vi "SynthHD_2_0a.vi"() -> ()   [LabVIEW 2012]
uses:
  Tab1.ctl
  <vilib>/Instr/_visa.llb/VISA Flush IO Buffer Mask.ctl
  <vilib>/Utility/file.llb/Read From Spreadsheet File (DBL).vi
  <vilib>/Utility/file.llb/Write To Spreadsheet File (DBL).vi
panel:
  out "RFOnB2":bool
  out "RFOnA2":bool
  out "Level B 2":bool
  out "Level A 2":bool
  in  "Modon":bool
  in  "Sync":bool
  out "POWER dBm B":dbl min=-100.0 max=24.0 step=1.0 format="%.2g"
  out "POWER dBm A":dbl min=-100.0 max=24.0 step=1.0 format="%.2g"
  out "RF  FREQUENCY MHz  B":dbl=1000.0 min=54.0 max=13900.0 step=1.0 format="%.7g"
  out "RF  FREQUENCY MHz A":dbl=1000.0 min=54.0 max=13900.0 step=1.0 format="%.7g"
  out "Amp Delta A -B":dbl format="%.2g"
  out "Freq Delta A-B":dbl format="%.7f"
  out "Device Under Control":string
  in  "AKNR":bool
  in  "PKNR":bool
  in  "FKNR":bool
  out "Channel":string="A"
  in  "ChSt":bool=TRUE
  out "COM Error":bool
  in  "Serial Port Select":refnum<visa-resource-name>="COM3"
  in  "stop":bool
  in  "Main Tab":T1
  in  "adn":bool
  in  "aup":bool
  in  "pdn":bool
  in  "pup":bool
  in  "fdn":bool
  in  "fup":bool
  out "Level":bool
  in  "Power Step Size":i32(ring)=3 items=["0.01dB", "0.05dB", "0.1 dB", "0.5 dB", "1.0 dB", "5.0 dB", "10.0 dB"]
  in  "RF  FREQUENCY MHz":dbl=1000.0 min=53.0 max=13999.999 step=1.0 format="%.7g"
  in  "Freqkn":i8(knob)=1 scale=1.0..20.0
  in  "Phasekn":i8(knob)=1 scale=1.0..20.0
  in  "PHASE Degrees":dbl min=0.0 max=360.0 step=1.0 format="%.2g"
  in  "POWER dBm":dbl min=-75.0 max=20.0 step=1.0 format="%.2g"
  in  "Powerkn":i8(knob)=1 scale=1.0..20.0
  in  "Frequency Step Size":i32(ring)=7 items=["0.1Hz", "1Hz", "10Hz", "100Hz", "1KHz", "10KHz", "100KHz", "1MHz", "10MHz", "100MHz", "1GHz"]
  in  "Phase Step Size":i32(ring)=6 items=["0.01 Degree", "0.05 Degree", "0.1 Degree", "0.5 Degree", "1 Degree", "5 Degree", "10 Degree", "90 Degree", "180 Degree"]
  in  "RF On":bool=TRUE
  in  "ChLock":bool
  in  "Sweep":enum32{"Linear", "List"}(tab)
  in  "Leveling":bool
  in  "Start Frequency":dbl=54.0 min=54.0 max=13900.0 step=0.001 format="%7.7f"
  in  "Step Size MHz":dbl=50.0 min=1e-07 max=13800.0 step=0.001 format="%.7f"
  in  "Stop Frequency":dbl=4000.0 min=54.0 max=13900.0 step=0.001 format="%7.7f"
  in  "Start Amplitude":dbl=22.0 min=-80.0 max=22.0 step=0.01 format="%7.2f"
  in  "Stop Amplitude":dbl=22.0 min=-80.0 max=22.0 step=0.01 format="%7.2f"
  out "Number\nof Points":u16
  out "Time per\nSweep (mS)":dbl format="%#.6g"
  in  "Read Table\nFrom File":bool
  in  "Save Table\nTo File":bool
  in  "Table RAM to\nTable NVROM":bool
  in  "Send Table\nTo RAM":bool
  in  "Sweep Table":dbl[][](array[numeric]) format="%#.6f"
  in  "Read Table\nFrom Device":bool
  in  "sweepdiff":bool
  in  "Sweep\nOnce":bool
  in  "Sweep\nContinuously":bool
  in  "sweepdir":bool
  in  "Differential Freq":dbl=54.0 min=-13800.0 max=13800.0 step=0.001 format="%7.7f"
  in  "Step Time (mS)":dbl=4.0 min=4.0 max=10000.0 step=0.001 format="%.3f"
  out "Swpc":string
  in  "Mod Tab":enum32{"PULSE Amplitude", "AM", "FM"}(tab)
  in  "Dual Channel Mode":bool
  in  "Send Pulse\nBurst":bool
  out "Duration (uS)":dbl
  in  "Continuous\nPM":bool
  in  "# of Pulses in Burst":u16=100 min=1 max=65500 step=1 format="%#.5f"
  in  "Off Time (uS)":u32=10 min=2 max=10000000 step=1
  in  "On Time (uS)":u32=1 max=10000000 step=1
  out "Pulsech":string
  in  "Invert\nPulse":bool
  in  "Read AM":bool
  out "Samples/Cycle":u8
  in  "Save AM to ROM":bool
  out "AMch":string
  in  "AM Freq (Hz)":dbl=500.0 min=1.0 max=5000.0 step=1.0 format="%.2f"
  out "Actual Freq (Hz)":dbl
  in  "Peak Power(dBm)":dbl=15.0 min=-74.9 max=20.0 step=0.01 format="%.2f"
  in  "Minimum Power (dBm)":dbl=15.0 min=-74.9 max=20.0 step=0.01 format="%.2f"
  in  "Continuous AM":bool
  in  "Wave Shape":u8(ring) items=["Sine", "Ramp", "Triangle"]
  out "Waveform":dbl[](graph)
  in  "Linear in?":u8(ring) items=["Linear in dB", "Linear in Volts"]
  in  "AM Samples in Burst":u16=100 min=1 max=5000 step=1 format="%#.5f"
  in  "FM Rate (Hz)":u16=500 min=1 max=5000 step=1
  in  "FM Deviation (+/- Hz)":u32=500 min=10 step=1
  in  "Continuous FM":bool
  in  "FM Samples in Burst":u16=100 min=1 max=65500 step=1 format="%#.5f"
  out "FMch":string
  in  "FM Function":u8(ring) items=["Sine", "Chirp"]
  out "FM Samples / Cycle":u16
  out "Specific Instructions":string
  in  "Trigger":i32(ring) items=["No Triggers", "Full Frequency Sweep", "Single Sweep Step", "Stop All", "Digital RF On/Off", "Remove Interrupts", "Reserved 1", "Reserved 2", "Ext AM Modulation", "Ext FM Modulation"]
  in  "Read Registers":bool
  in  "Read Settings\nFrom SynthHD":bool
  out "read buffer":string
  out "Hex buf":string
  in  "MUX Out Select":u8(ring)=6 items=["HiZ", "Vdd", "GND", "R Divider", "N Divider", "An Lock Det", "Dig Lock Det"]
  in  "PLL ICP":u8=4 max=15 step=1 format="%02d"
  out "HW Version":string
  in  "Get Phase\nLock Status":bool
  out "FW Version":string
  in  "Read\nVersion":bool
  in  "Save Settings\nto ROM":bool
  in  "Get\nTemperature":bool
  out "Temperature":string
  in  "Fundamental\nFeedback Mode":bool
  out "Lock":bool
  in  "MTLD":bool
  in  "Re-Init Settings\nto Default":bool
  in  "Reference Select":u8(ring)=1 items=["External", "Internal 27MHz", "Internal 10MHz"]
  in  "Reference (MHz)":dbl=27.0 min=5.0 max=111.0 step=0.001 format="%7.6g"
  # "A"
  # "B"
  # "v2.0a"
  # "Windfreak Technologies"
  # "A"
  # "B"
  # "Tab selection dictates sweep mode"
  # "Step"
  # "Freq(MHz)"
  # "Level(dBm)"
  # "Burst"
  # "Widest FM Deviation+/- \n54-106.25MHz = 160KHz\n-212.5MHz        = 312KHz\n-425.0MHz        = 625KHz\n-850.0MHz      = 1.25MHz\n-1700MHz         = 2.5MHz\n-3400MHz            = 5MHz\n-6800MHz          = 10MHz\n-13600MHz        = 20MHz"
  # "Digital Trigger 0V to +3.3V only.\nAnalog Input 0V to 1.2V only.\nTrigger has ~35K ohm pullup\nfor both modes."
  # "C"
  # "Windfreak Technologies, LLC 2015"
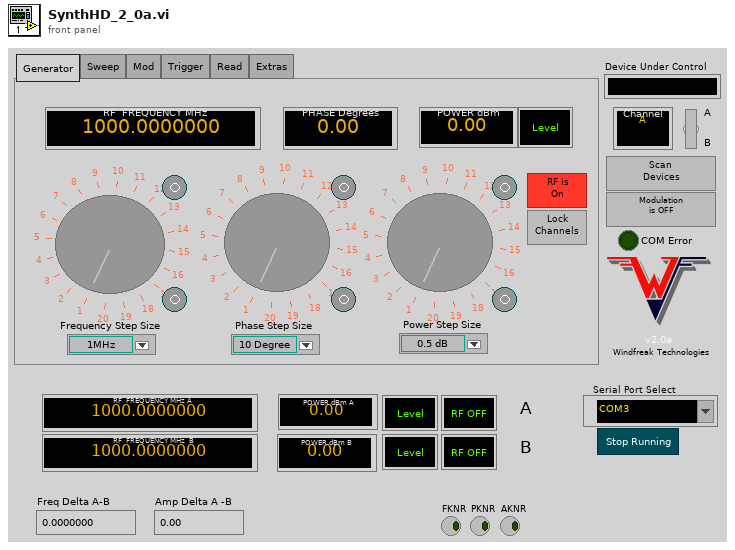
[diagram p1: front panel]
types:
  T1 = typedef "Tab1.ctl" = enum32{"Generator", "Sweep", "Mod", "Trigger", "Read", "Extras"}
  T2 = enum8{"Enabled", "Disabled", "Disabled and Grayed Out"}
  T3 = cluster{"[0]":dbl, "[1]":dbl, "[2]":dbl, "[3]":dbl, "[4]":dbl, "[5]":dbl, "[6]":dbl, "[7]":dbl, "[8]":dbl, "[9]":dbl, "[10]":dbl, "[11]":dbl, "[12]":dbl, "[13]":dbl, "[14]":dbl, "[15]":dbl, "[16]":dbl, "[17]":dbl, "[18]":dbl, "[19]":dbl, "[20]":dbl, "[21]":dbl, "[22]":dbl, "[23]":dbl, "[24]":dbl, "[25]":dbl, "[26]":dbl, "[27]":dbl, "[28]":dbl, "[29]":dbl, "[30]":dbl, "[31]":dbl, "[32]":dbl, "[33]":dbl, "[34]":dbl, "[35]":dbl, "[36]":dbl, "[37]":dbl, "[38]":dbl, "[39]":dbl, "[40]":dbl, "[41]":dbl}
  T4 = typedef "VISA Flush IO Buffer Mask.ctl" = u16
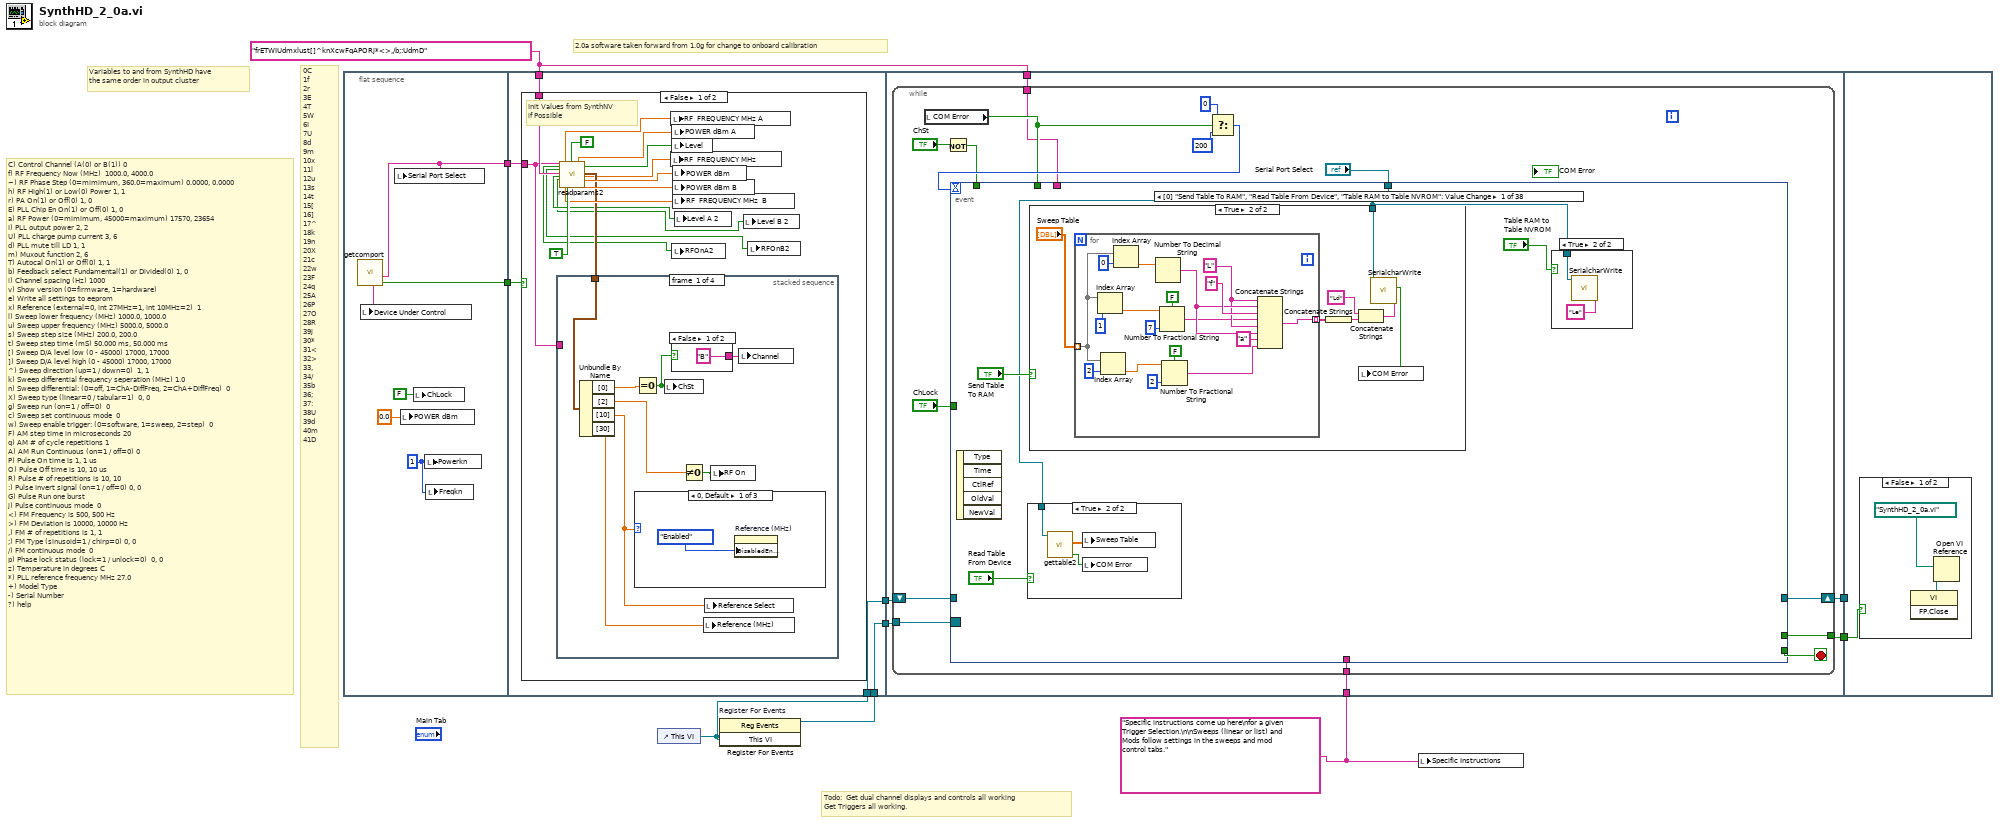
[diagram p0: block diagram]
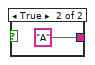
[diagram p2: hidden frame]
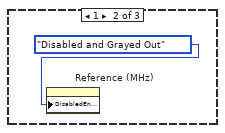
[diagram p3: hidden frame]
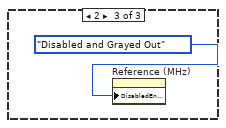
[diagram p4: hidden frame]
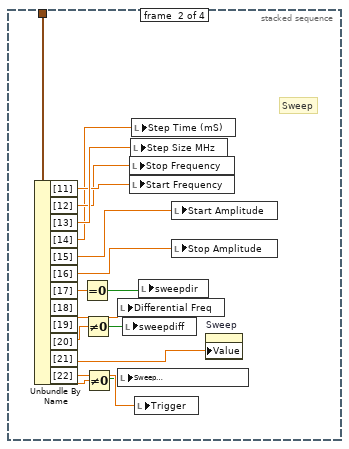
[diagram p5: hidden frame]
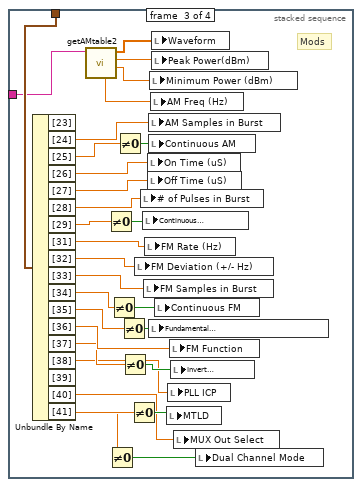
[diagram p6: hidden frame]
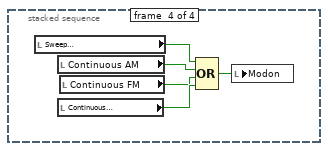
[diagram p7: hidden frame]
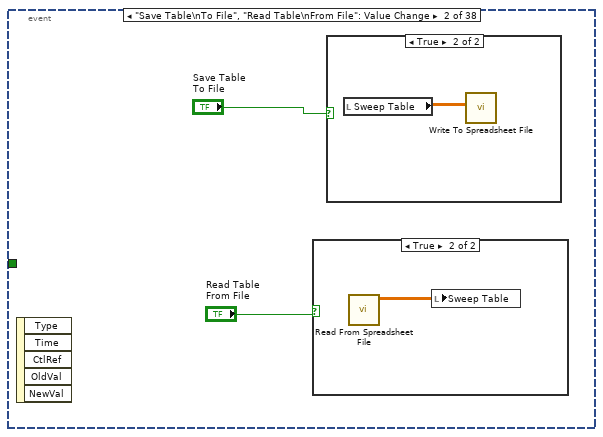
[diagram p12: hidden frame]
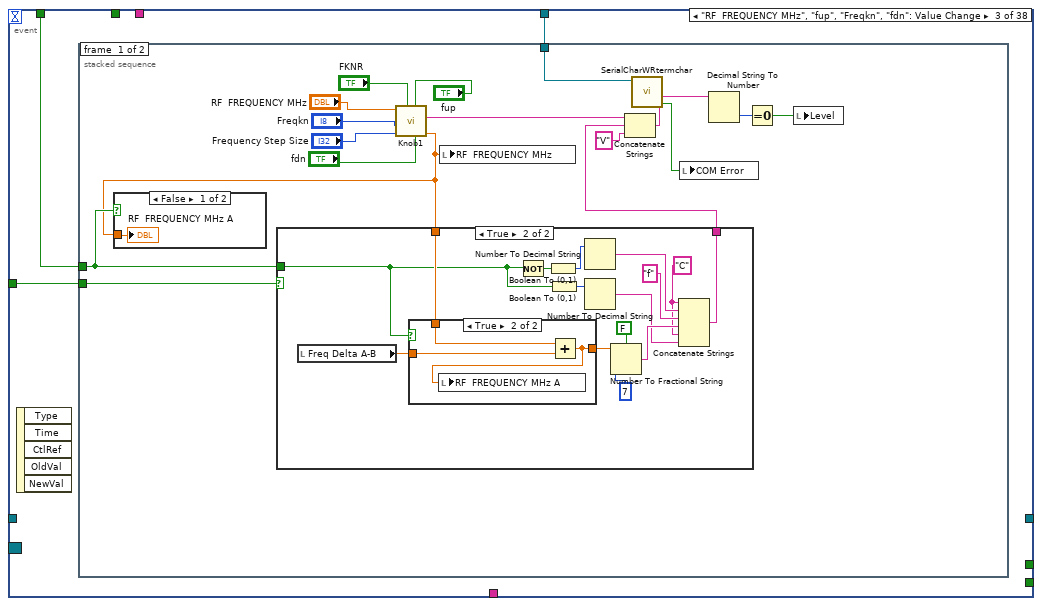
[diagram p15: hidden frame]
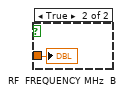
[diagram p16: hidden frame]
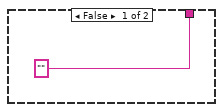
[diagram p17: hidden frame]
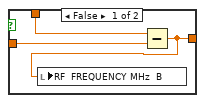
[diagram p18: hidden frame]
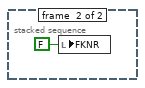
[diagram p19: hidden frame]
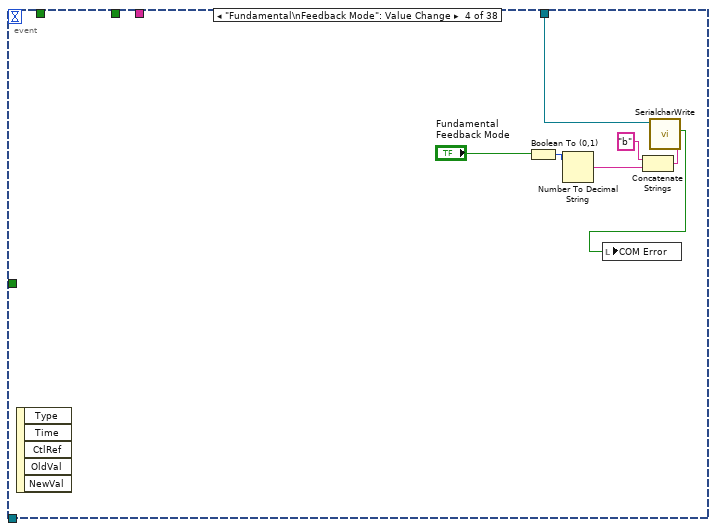
[diagram p20: hidden frame]
diagram:
  w1 = "Specific instructions come up here\nfor a given Trigger Selection.\n\nSweeps (linear or list) and Mods follow settings in the sweeps and mod control tabs." ("message")
  w4 = "frETWIUdmxlust[]^knXcwFqAPORj*<>,/b;:UdmD" ("var query")
  # "Todo:  Get dual channel displays and controls all working\nGet Triggers all working."
  # "2.0a software taken forward from 1.0g for change to onboard calibration"
  # "C) Control Channel (A(0) or B(1)) 0\nf) RF Frequency Now (MHz)  1000.0, 4000.0\n~) RF Phase Step (0=mimimum, 360.0=maximum) 0.0000, 0.0000\nh) RF High(1) or Low(0) Power 1, 1\nr) PA On(1) or Off(0) 1, 0\nE) PLL Chip En On(1) or Off(0) 1, 0\na) RF Power (0=mimimum, 45000=maximum) 17570, 23654\nI) PLL output power 2, 2\nU) PLL charge pump current 3, 6\nd) PLL mute till LD 1, 1\nm) Muxout function 2, 6\nT) Autocal On(1) or Off(0) 1, 1\nb) Feedback select Fundamental(1) or Divided(0) 1, 0\ni) Channel spacing (Hz) 1000\nv) Show version (0=firmware, 1=hardware)\ne) Write all settings to eeprom\nx) Reference (external=0, int 27MHz=1, int 10MHz=2)  1\nl) Sweep lower frequency (MHz) 1000.0, 1000.0\nu) Sweep upper frequency (MHz) 5000.0, 5000.0\ns) Sweep step size (MHz) 200.0, 200.0\nt) Sweep step time (mS) 50.000 ms, 50.000 ms\n[) Sweep D/A level low (0 - 45000) 17000, 17000\n]) Sweep D/A level high (0 - 45000) 17000, 17000\n^) Sweep direction (up=1 / down=0)  1, 1\nk) Sweep differential frequency seperation (MHz) 1.0\nn) Sweep differential: (0=off, 1=ChA-DiffFreq, 2=ChA+DiffFreq)  0\nX) Sweep type (linear=0 / tabular=1)  0, 0\ng) Sweep run (on=1 / off=0)  0\nc) Sweep set continuous mode  0\nw) Sweep enable trigger: (0=software, 1=sweep, 2=step)  0\nF) AM step time in microseconds 20\nq) AM # of cycle repetitions 1\nA) AM Run Continuous (on=1 / off=0) 0\nP) Pulse On time is 1, 1 us\nO) Pulse Off time is 10, 10 us\nR) Pulse # of repetitions is 10, 10\n:) Pulse Invert signal (on=1 / off=0) 0, 0\nG) Pulse Run one burst\nj) Pulse continuous mode  0\n<) FM Frequency is 500, 500 Hz\n>) FM Deviation is 10000, 10000 Hz\n,) FM # of repetitions is 1, 1\n;) FM Type (sinusoid=1 / chirp=0) 0, 0\n/) FM continuous mode  0\np) Phase lock status (lock=1 / unlock=0)  0, 0\nz) Temperature in degrees C\n*) PLL reference frequency MHz 27.0\n+) Model Type\n-) Serial Number  \n?) help"
  # "0C\n1f\n2r\n3E\n4T\n5W\n6I\n7U\n8d\n9m\n10x\n11l\n12u\n13s\n14t\n15[\n16]\n17^\n18k\n19n\n20X\n21c\n22w\n23F\n24q\n25A\n26P\n27O\n28R\n39j\n30*\n31<\n32>\n33,\n34/\n35b\n36;\n37:\n38U\n39d\n40m\n41D"
  # "Variables to and from SynthHD have \nthe same order in output cluster"
  n1 = flat-sequence {
    tunnel: [w16] -> w10
    tunnel: [w15] -> w9
    tunnel: w10 -> [w21]
    tunnel: w9 -> [w20]
    tunnel: [w18] -> w8
    tunnel: [w17] -> w7
    tunnel: w4 -> [w19]
    tunnel: w3 -> [w18]
    tunnel: w2 -> [w17]
    tunnel: w8 -> [w106]
    tunnel: w7 -> [w107]
    tunnel: [w105] -> w6
    tunnel: [w104] -> w5
    tunnel: w4 -> [w103]
    tunnel: w1 -> [w102]
    tunnel: w6 -> [_]
    tunnel: w5 -> [w811]
    frame #0 {
      w13 = i8 1 ("Powerkn")
      n2 = call "getcomport.vi"() -> ("No Devices"=w16:bool, "Port"=w15:string, "Device"=w14:string)  [unwired: 9 in]
      n3 = local write "Device Under Control"(w14) -> ()
      n4 = local write "Serial Port Select"(w15) -> ()
      n5 = local write "POWER dBm"(0.0 ("Power")) -> ()
      n6 = local write "ChLock"(FALSE ("ChLock")) -> ()
      n7 = local write "Powerkn"(w13) -> ()
      n8 = local write "Freqkn"(w13) -> ()
    }
    frame #1 {
      n9 = case shown="False" w21 {
        tunnel: w20 -> [w27 _]
        tunnel: w19 -> [w37 _]
        frame False {
          # "Init Values from SynthNV\nif Possible"
          n10 = call "readparams2.vi"("Port In"=w27, "var query"=w37, "Get F&A"=TRUE, "Prog Chan?"=FALSE) -> ("RFonA"=w23:bool, "RFonB"=w22:bool, "LevA"=w25:bool, "LevB"=w24:bool, "FchA"=w35:dbl, "FchB"=w32:dbl, "AdBm"=w34:dbl, "BdBm"=w33:dbl, "NowLevel"=w31:bool, "cluster"=w28:T3, "NowFreq"=w26:dbl, "NowdBm"=w30:dbl)  [unwired: 9 in, 3 out]
          n11 = stacked-sequence {
            tunnel: w28 -> [w42 w66 w96 _]
            tunnel: w27 -> [_ _ w84 _]
            frame #0 {
              n12 = Unbundle By Name(w42) -> ("[0]"=w45:dbl, "[2]"=w44:dbl, "[10]"=w41:dbl, "[30]"=w40:dbl)
              n13 = Equal To 0?(x=w45) -> (x = 0?=w38:bool)
              n14 = case shown="0, Default" w41 {
                frame 0, Default {
                  n15 = property on="Reference (MHz)" class="DigNum (strict)"("DisabledEnum"=T2."Enabled" ("Disabled")) -> ()  [unwired: 2 in, 2 out]
                }
                frame 1 {
                  n16 = property on="Reference (MHz)" class="DigNum (strict)"("DisabledEnum"=T2."Disabled and Grayed Out" ("Disabled")) -> ()  [unwired: 2 in, 2 out]
                }
                frame 2 {
                  n17 = property on="Reference (MHz)" class="DigNum (strict)"("DisabledEnum"=T2."Disabled and Grayed Out" ("Disabled")) -> ()  [unwired: 2 in, 2 out]
                }
              }
              n18 = local write "ChSt"(w38) -> ()
              n19 = case shown="False" w38 {
                tunnel: ["B" ("Channel") "A" ("Channel")] -> w43
                frame False {
                }
                frame True {
                }
              }
              n20 = Not Equal To 0?(x=w44) -> (x != 0?=w39:bool)
              n21 = local write "Reference (MHz)"(w40) -> ()
              n22 = local write "Reference Select"(w41) -> ()
              n23 = local write "RF On"(w39) -> ()
              n24 = local write "Channel"(w43) -> ()
            }
            frame #1 {
              # "Sweep"
              n25 = Unbundle By Name(w66) -> ("[11]"=w56:dbl, "[12]"=w55:dbl, "[13]"=w65:dbl, "[14]"=w54:dbl, "[15]"=w52:dbl, "[16]"=w51:dbl, "[17]"=w64:dbl, "[18]"=w62:dbl, "[19]"=w61:dbl, "[20]"=w57:dbl, "[21]"=w53:dbl, "[22]"=w59:dbl)
              n26 = Equal To 0?(x=w64) -> (x = 0?=w63:bool)
              n27 = Not Equal To 0?(x=w61) -> (x != 0?=w60:bool)
              n28 = Not Equal To 0?(x=w53) -> (x != 0?=w58:bool)
              n29 = local write "Differential Freq"(w62) -> ()
              n30 = local write "Sweep\nContinuously"(w58) -> ()
              n31 = local write "sweepdiff"(w60) -> ()
              n32 = local write "Stop Frequency"(w55) -> ()
              n33 = local write "Start Frequency"(w56) -> ()
              n34 = local write "Step Size MHz"(w65) -> ()
              n35 = local write "Step Time (mS)"(w54) -> ()
              n36 = local write "Trigger"(w59) -> ()
              n37 = local write "sweepdir"(w63) -> ()
              n38 = local write "Start Amplitude"(w52) -> ()
              n39 = local write "Stop Amplitude"(w51) -> ()
              n40 = property on="Sweep" class="TabCtl (strict)"("Value"=w57) -> ()  [unwired: 2 in, 2 out]
            }
            frame #2 {
              # "Mods"
              n41 = Unbundle By Name(w96) -> ("[24]"=w81:dbl, "[25]"=w93:dbl, "[26]"=w92:dbl, "[27]"=w91:dbl, "[28]"=w90:dbl, "[29]"=w89:dbl, "[31]"=w83:dbl, "[32]"=w82:dbl, "[33]"=w79:dbl, "[34]"=w80:dbl, "[35]"=w76:dbl, "[36]"=w75:dbl, "[37]"=w73:dbl, "[38]"=w72:dbl, "[39]"=w70:dbl, "[40]"=w69:dbl, "[41]"=w68:dbl)  [unwired: 1 out]
              n42 = call "getAMtable2.vi"("Serial Port Select"=w84) -> ("Min dB"=w85:dbl, "Max dB"=w86:dbl, "Waveform Graph"=w87:dbl[], "AM Freq Hz"=w88:dbl)  [unwired: 5 in, 2 out]
              n43 = Not Equal To 0?(x=w89) -> (x != 0?=w94:bool)
              n44 = Not Equal To 0?(x=w68) -> (x != 0?=w67:bool)
              n45 = Not Equal To 0?(x=w80) -> (x != 0?=w78:bool)
              n46 = Not Equal To 0?(x=w93) -> (x != 0?=w95:bool)
              n47 = Not Equal To 0?(x=w76) -> (x != 0?=w77:bool)
              n48 = Not Equal To 0?(x=w73) -> (x != 0?=w74:bool)
              n49 = Not Equal To 0?(x=w70) -> (x != 0?=w71:bool)
              n50 = local write "FM Deviation (+/- Hz)"(w82) -> ()
              n51 = local write "# of Pulses in Burst"(w90) -> ()
              n52 = local write "Continuous\nPM"(w94) -> ()
              n53 = local write "FM Samples in Burst"(w79) -> ()
              n54 = local write "FM Rate (Hz)"(w83) -> ()
              n55 = local write "On Time (uS)"(w92) -> ()
              n56 = local write "Off Time (uS)"(w91) -> ()
              n57 = local write "AM Samples in Burst"(w81) -> ()
              n58 = local write "Continuous AM"(w95) -> ()
              n59 = local write "Fundamental\nFeedback Mode"(w77) -> ()
              n60 = local write "Minimum Power (dBm)"(w85) -> ()
              n61 = local write "AM Freq (Hz)"(w88) -> ()
              n62 = local write "Waveform"(w87) -> ()
              n63 = local write "Peak Power(dBm)"(w86) -> ()
              n64 = local write "Continuous FM"(w78) -> ()
              n65 = local write "MTLD"(w71) -> ()
              n66 = local write "PLL ICP"(w72) -> ()
              n67 = local write "FM Function"(w75) -> ()
              n68 = local write "Invert\nPulse"(w74) -> ()
              n69 = local write "MUX Out Select"(w69) -> ()
              n70 = local write "Dual Channel Mode"(w67) -> ()
            }
            frame #3 {
              n71 = local read "Sweep\nContinuously"() -> (w98:bool)
              n72 = local read "Continuous AM"() -> (w99:bool)
              n73 = local read "Continuous\nPM"() -> (w101:bool)
              n74 = local read "Continuous FM"() -> (w100:bool)
              n75 = Compound Arithmetic op=OR(w98, w99, w100, w101) -> (w97:bool)
              n76 = local write "Modon"(w97) -> ()
            }
          }
          n77 = local write "RF  FREQUENCY MHz A"(w35) -> ()
          n78 = local write "RF  FREQUENCY MHz"(w26) -> ()
          n79 = local write "POWER dBm A"(w34) -> ()
          n80 = local write "Level"(w31) -> ()
          n81 = local write "RFOnA2"(w23) -> ()
          n82 = local write "POWER dBm"(w30) -> ()
          n83 = local write "POWER dBm B"(w33) -> ()
          n84 = local write "RF  FREQUENCY MHz  B"(w32) -> ()
          n85 = local write "Level A 2"(w25) -> ()
          n86 = local write "Level B 2"(w24) -> ()
          n87 = local write "RFOnB2"(w22) -> ()
        }
        frame True {
        }
      }
    }
    frame #2 {
      n88 = while {
        shift-right: [w118] -> w105
        shift-left: w107 -> [w120]
        tunnel: w106 -> [w119]
        tunnel: [w117] -> w104
        tunnel: w103 -> [w112]
        tunnel: w102 -> [w108]
        stop <- w121 stop-if-true
        n89 = local read "COM Error"() -> (w113:bool)
        n90 = Not(x="ChSt") -> (.not. x?=w110:bool)
        n91 = Select(t=0, s=w113, f=200) -> (s? t:f=w114:i32)
        n92 = event shown="[0] \"Send Table To RAM\", \"Read Table From Device\", \"Table RAM to Table NVROM\": Value Change" {
          selector: w119 -> [_ _ _ _ _ _ _ _ _ _ _ _ _ _ _ _ _ _ _ _ _ _ _ _ _ _ _ _ _ _ _ _ _ _ _ _ _ _]
          dyn-events: _ -> [_ _ _ _ _ _ _ _ _ _ _ _ _ _ _ _ _ _ _ _ _ _ _ _ _ _ _ _ _ _ _ _ _ _ _ _ _ _]
          timeout: w114 -> [_ _ _ _ _ _ _ _ _ _ _ _ _ _ _ _ _ _ _ _ _ _ _ _ _ _ _ _ _ _ _ _ _ _ _ _ _ _]
          tunnel: "Serial Port Select" -> [w123 _ w163 w207 w214 w254 w326 _ w374 w403 w425 w437 w471 w479 w496 w509 w524 w539 w542 w544 w549 w552 w560 w564 w585 w589 w594 w601 w718 w751 w764 w771 w775 _ _ w784 w790 w800]
          tunnel: [_ _ _ _ _ _ _ _ _ _ _ _ _ _ _ _ _ _ _ _ _ _ _ _ _ _ _ _ _ _ _ _ _ "stop" w781 _ _ _] -> w121
          tunnel: w120 -> [_ _ _ _ _ _ _ _ _ _ _ _ _ _ _ _ _ _ _ _ _ _ _ _ _ _ _ _ _ _ _ _ _ _ w780 _ _ _]
          tunnel: [_ _ _ _ _ _ _ _ _ _ _ _ _ _ _ _ _ _ _ _ _ _ _ _ _ _ _ _ _ _ _ _ _ _ w780 _ _ _] -> w118
          tunnel: [_ _ _ _ _ _ _ _ _ _ _ _ _ _ _ _ _ _ _ _ _ _ _ _ _ _ _ _ _ _ _ _ _ "stop" _ _ _ _] -> w117
          tunnel: w113 -> [_ _ _ _ _ _ _ _ _ _ _ _ _ _ _ _ _ _ _ _ _ _ _ _ _ _ _ _ _ _ _ _ _ _ _ w783 _ _]
          tunnel: w112 -> [_ _ _ _ _ _ _ _ _ _ _ _ _ _ _ _ _ _ _ _ _ _ _ _ _ _ _ w602 _ _ _ _ _ _ _ _ _ _]
          tunnel: w110 -> [_ _ w162 _ _ w253 w319 _ _ _ _ w435 w463 _ w489 _ w518 _ _ _ _ _ _ _ _ _ _ w600 _ _ w755 _ _ _ _ _ _ _]
          tunnel: "ChLock" -> [_ _ w161 _ _ w252 _ _ _ _ _ _ _ _ _ _ _ _ _ _ _ _ _ _ _ _ _ _ _ _ _ _ _ _ _ _ _ _]
          tunnel: w108 -> [_ _ _ _ _ _ _ _ _ w400 _ _ _ _ _ _ _ _ _ _ _ _ _ _ _ _ _ _ _ _ _ _ _ _ _ _ _ _]
          event "Send Table\nTo RAM", "Read Table\nFrom Device", "Table RAM to\nTable NVROM": Value Change {
            n93 = event-data() -> ()  [unwired: 1 in, 5 out]
            n94 = case shown="True" "Read Table\nFrom Device" {
              tunnel: w123 -> [_ w131]
              frame False {
              }
              frame True {
                n95 = call "gettable2.vi"("Serial Port Select"=w131) -> ("COM Error"=w130:bool, "Sweep Table"=w129:dbl[][])  [unwired: 9 in]
                n96 = local write "Sweep Table"(w129) -> ()
                n97 = local write "COM Error"(w130) -> ()
              }
            }
            n98 = case shown="True" "Send Table\nTo RAM" {
              tunnel: w123 -> [_ w137]
              frame False {
              }
              frame True {
                n99 = for {
                  tunnel: "Sweep Table" -> [w145] mode=indexing
                  tunnel: [w151] -> w132 mode=indexing
                  w148 = "L" ("string")
                  n100 = Index Array(array=w145, index=1) -> (element=w144:dbl)
                  n101 = Index Array(array=w145, index=2) -> (element=w140:dbl)
                  n102 = Index Array(array=w145, index=0) -> (element=w149:dbl)
                  n103 = Number To Decimal String(number=w149) -> (decimal integer string=w152:string)  [unwired: 1 in]
                  n104 = Number To Fractional String(use system decimal point (T)=FALSE, number=w144, precision (6)=i16 7) -> (F-format string=w147:string)  [unwired: 1 in]
                  n105 = Number To Fractional String(use system decimal point (T)=FALSE, number=w140, precision (6)=i16 2) -> (F-format string=w139:string)  [unwired: 1 in]
                  n106 = Concatenate Strings(w148, w152, "f" ("string"), w147, w148, w152, "a" ("string"), w139) -> (w151:string)
                }
                n107 = Concatenate Strings(w132) -> (w135:string)
                n108 = Concatenate Strings("Ld" ("string"), w135) -> (w133:string)
                n109 = call "SerialcharWrite.vi"("VISA resource name"=w137, "write buffer"=w133) -> ("ComError"=w136:bool)  [unwired: 8 in]
                n110 = local write "COM Error"(w136) -> ()
              }
            }
            n111 = case shown="True" "Table RAM to\nTable NVROM" {
              tunnel: w123 -> [_ w128]
              frame False {
              }
              frame True {
                n112 = call "SerialcharWrite.vi"("VISA resource name"=w128, "write buffer"="Le") -> ()  [unwired: 8 in, 1 out]
              }
            }
          }
          event "Save Table\nTo File", "Read Table\nFrom File": Value Change {
            n113 = event-data() -> ()  [unwired: 1 in, 5 out]
            n114 = case shown="True" "Read Table\nFrom File" {
              frame False {
              }
              frame True {
                n115 = call-poly <vilib>:"Read From Spreadsheet File.vi"() -> ("all rows"=w159:dbl[][])  [unwired: 7 in, 4 out]
                n116 = local write "Sweep Table"(w159) -> ()
              }
            }
            n117 = case shown="True" "Save Table\nTo File" {
              frame False {
              }
              frame True {
                n118 = local read "Sweep Table"() -> (w160:dbl[][])
                n119 = call-poly <vilib>:"Write To Spreadsheet File.vi"("2D data"=w160) -> ()  [unwired: 7 in, 1 out]
              }
            }
          }
          event "RF  FREQUENCY MHz", "fup", "Freqkn", "fdn": Value Change {
            n120 = event-data() -> ()  [unwired: 1 in, 5 out]
            n121 = stacked-sequence {
              tunnel: w163 -> [w181 _]
              tunnel: w162 -> [w169 _]
              tunnel: w161 -> [w171 _]
              frame #0 {
                n122 = call "Knob1.vi"("Freqin"="RF  FREQUENCY MHz", "Knob"="Freqkn", "Frequency Step Size"="Frequency Step Size", "Reset"="FKNR", "fup"="fup", "fdn"="fdn") -> ("freqcommand"=w176:string, "freqout"=w168:dbl)  [unwired: 3 in]
                n123 = case shown="False" w169 {
                  tunnel: w168 -> [w182 w183]
                  frame False {
                    "RF  FREQUENCY MHz A" <- w182
                  }
                  frame True {
                    "RF  FREQUENCY MHz  B" <- w183
                  }
                }
                n124 = case shown="True" w171 {
                  tunnel: ["" ("string") w199] -> w170
                  tunnel: w168 -> [_ w190]
                  tunnel: w169 -> [_ w187]
                  frame False {
                  }
                  frame True {
                    w186 = "C" ("string")
                    n125 = local read "Freq Delta A-B"() -> (w192:dbl)
                    n126 = case shown="True" w187 {
                      tunnel: w190 -> [w201 w205]
                      tunnel: [w200 w203] -> w189
                      tunnel: w192 -> [w202 w204]
                      frame False {
                        n127 = Subtract(x=w201, y=w202) -> (x-y=w200:dbl)
                        n128 = local write "RF  FREQUENCY MHz  B"(w200) -> ()
                      }
                      frame True {
                        n129 = Add(x=w205, y=w204) -> (x+y=w203:dbl)
                        n130 = local write "RF  FREQUENCY MHz A"(w203) -> ()
                      }
                    }
                    n131 = Not(x=w187) -> (.not. x?=w188:bool)
                    n132 = Boolean To (0,1)(Boolean=w188) -> (0, 1=w194:i16)
                    n133 = Boolean To (0,1)(Boolean=w187) -> (0, 1=w193:i16)
                    n134 = Number To Decimal String(number=w194) -> (decimal integer string=w198:string)  [unwired: 1 in]
                    n135 = Number To Decimal String(number=w193) -> (decimal integer string=w185:string)  [unwired: 1 in]
                    n136 = Number To Fractional String(use system decimal point (T)=FALSE, number=w189, precision (6)=i16 7) -> (F-format string=w195:string)  [unwired: 1 in]
                    n137 = Concatenate Strings(w186, w198, "f" ("string"), w195, w186, w185) -> (w199:string)
                  }
                }
                n138 = local write "RF  FREQUENCY MHz"(w168) -> ()
                n139 = Concatenate Strings(w176, w170, "V" ("string")) -> (w179:string)
                n140 = call "SerialCharWRtermchar.vi"("VISA resource name"=w181, "write buffer"=w179) -> ("error?"=w180:bool, "read buffer"=w164:string)  [unwired: 6 in, 1 out]
                n141 = local write "COM Error"(w180) -> ()
                n142 = Decimal String To Number(string=w164) -> (number=w165:i32)  [unwired: 2 in, 1 out]
                n143 = Equal To 0?(x=w165) -> (x = 0?=w166:bool)
                n144 = local write "Level"(w166) -> ()
              }
              frame #1 {
                n145 = local write "FKNR"(FALSE ("Reset")) -> ()
              }
            }
          }
          event "Fundamental\nFeedback Mode": Value Change {
            n146 = event-data() -> ()  [unwired: 1 in, 5 out]
            n147 = Boolean To (0,1)(Boolean="Fundamental\nFeedback Mode") -> (0, 1=w211:i16)
            n148 = Number To Decimal String(number=w211) -> (decimal integer string=w209:string)  [unwired: 1 in]
            n149 = Concatenate Strings("b" ("element"), w209) -> (w212:string)
            n150 = call "SerialcharWrite.vi"("VISA resource name"=w207, "write buffer"=w212) -> ("ComError"=w210:bool)  [unwired: 8 in]
            n151 = local write "COM Error"(w210) -> ()
          }
          event "PHASE Degrees", "Phasekn", "pup", "pdn": Value Change {
            n152 = event-data() -> ()  [unwired: 1 in, 5 out]
            n153 = stacked-sequence {
              tunnel: w214 -> [w219 _]
              frame #0 {
                n154 = case shown="8" "Phase Step Size" {
                  tunnel: [0.01 0.05 0.1 0.5 1.0 5.0 10.0 90.0 180.0] -> w218
                  frame 0, Default {
                  }
                  frame 1 {
                  }
                  frame 2 {
                  }
                  frame 3 {
                  }
                  frame 4 {
                  }
                  frame 5 {
                  }
                  frame 6 {
                  }
                  frame 7 {
                  }
                  frame 8 {
                  }
                }
                n155 = call "Knobphase.vi"("Freqin"="PHASE Degrees", "Knob"="Phasekn", "Step Size"=w218, "Reset"="PKNR", "pup"="pup", "pdn"="pdn") -> ("Freqout"=w221:dbl, "Phase Pr Out"=w217:dbl)  [unwired: 3 in]
                n156 = Greater Or Equal?(x=w221, y=360.0) -> (x >= y?=w222:bool)
                n157 = case shown="False" w222 {
                  tunnel: w221 -> [w233 _]
                  tunnel: w218 -> [w234 _]
                  frame False {
                    n158 = Less?(x=w233, y=0.0) -> (x < y?=w235:bool)
                    n159 = case shown="False" w235 {
                      tunnel: w234 -> [_ w239]
                      tunnel: w233 -> [w237 _]
                      frame False {
                        n160 = local write "PHASE Degrees"(w237) -> ()
                      }
                      frame True {
                        n161 = Subtract(x=360.0 ("Phase Degrees"), y=w239) -> (x-y=w238:dbl)
                        n162 = local write "PHASE Degrees"(w238) -> ()
                      }
                    }
                  }
                  frame True {
                    n163 = local write "PHASE Degrees"(0.0 ("Phase Degrees")) -> ()
                  }
                }
                n164 = Number To Fractional String(use system decimal point (T)=FALSE, number=w217, precision (6)=i16 2) -> (F-format string=w228:string)  [unwired: 1 in]
                n165 = Concatenate Strings("~" ("element"), w228) -> (w230:string)
                n166 = call "SerialcharWrite.vi"("VISA resource name"=w219, "write buffer"=w230) -> ("ComError"=w231:bool)  [unwired: 8 in]
                n167 = local write "COM Error"(w231) -> ()
              }
              frame #1 {
                n168 = local write "PKNR"(FALSE ("PKNR")) -> ()
              }
            }
          }
          event "Powerkn", "POWER dBm", "aup", "adn": Value Change {
            n169 = event-data() -> ()  [unwired: 1 in, 5 out]
            n170 = stacked-sequence {
              tunnel: w254 -> [w274 _]
              tunnel: w253 -> [w256 _]
              tunnel: w252 -> [w266 _]
              frame #0 {
                # "Sweep Leveling"
                # "write to VGA"
                n171 = case shown="3" "Power Step Size" {
                  tunnel: [0.01 0.05 0.1 0.5 1.0 5.0 10.0] -> w272
                  frame 0, Default {
                  }
                  frame 1 {
                  }
                  frame 2 {
                  }
                  frame 3 {
                  }
                  frame 4 {
                  }
                  frame 5 {
                  }
                  frame 6 {
                  }
                }
                n172 = call "Knob3.vi"("PwrIn"="POWER dBm", "Knob"="Powerkn", "Step Size"=w272, "Reset"="AKNR", "aup"="aup", "adn"="adn") -> ("PwrSet"=w261:string, "PwrOut"=w262:dbl)  [unwired: 3 in]
                n173 = case shown="True" w266 {
                  tunnel: ["" ("string") w303] -> w265
                  tunnel: w256 -> [_ w296]
                  tunnel: w262 -> [_ w299]
                  frame False {
                  }
                  frame True {
                    w291 = "C" ("string")
                    n174 = local read "Amp Delta A -B"() -> (w300:dbl)
                    n175 = case shown="True" w296 {
                      tunnel: [w304 w307] -> w295
                      tunnel: w300 -> [w306 w309]
                      tunnel: w299 -> [w305 w308]
                      frame False {
                        n176 = Subtract(x=w305, y=w306) -> (x-y=w304:dbl)
                        n177 = local write "POWER dBm B"(w304) -> ()
                      }
                      frame True {
                        n178 = Add(x=w308, y=w309) -> (x+y=w307:dbl)
                        n179 = local write "POWER dBm A"(w307) -> ()
                      }
                    }
                    n180 = Not(x=w296) -> (.not. x?=w297:bool)
                    n181 = Boolean To (0,1)(Boolean=w297) -> (0, 1=w302:i16)
                    n182 = Boolean To (0,1)(Boolean=w296) -> (0, 1=w301:i16)
                    n183 = Number To Decimal String(number=w302) -> (decimal integer string=w290:string)  [unwired: 1 in]
                    n184 = Number To Decimal String(number=w301) -> (decimal integer string=w298:string)  [unwired: 1 in]
                    n185 = Number To Fractional String(use system decimal point (T)=FALSE, number=w295, precision (6)=i16 2) -> (F-format string=w292:string)  [unwired: 1 in]
                    n186 = Concatenate Strings(w291, w290, "W" ("string"), w292, w291, w298) -> (w303:string)
                  }
                }
                n187 = case shown="True" w256 {
                  tunnel: w262 -> [w286 w287]
                  frame False {
                    "POWER dBm A" <- w286
                  }
                  frame True {
                    "POWER dBm B" <- w287
                  }
                }
                n188 = local write "POWER dBm"(w262) -> ()
                n189 = local read "Leveling"() -> (w264:bool)
                n190 = case shown="True" w264 {
                  tunnel: ["" ("string") w280] -> w263
                  tunnel: w261 -> [_ w284]
                  tunnel: w262 -> [_ w279]
                  frame False {
                  }
                  frame True {
                    n191 = String Subset(string=w284, offset (0)=1) -> (substring=w282:string)  [unwired: 1 in]
                    n192 = local write "Start Amplitude"(w279) -> ()
                    n193 = local write "Stop Amplitude"(w279) -> ()
                    n194 = Concatenate Strings("[" ("string"), w282, "]" ("string"), w282) -> (w280:string)
                  }
                }
                n195 = Concatenate Strings(w261, w265, w263, "V" ("string")) -> (w260:string)
                n196 = call "SerialCharWRtermchar.vi"("VISA resource name"=w274, "write buffer"=w260) -> ("error?"=w275:bool, "read buffer"=w258:string)  [unwired: 6 in, 1 out]
                n197 = Decimal String To Number(string=w258) -> (number=w257:i32)  [unwired: 2 in, 1 out]
                n198 = local write "COM Error"(w275) -> ()
                n199 = Equal To 0?(x=w257) -> (x = 0?=w255:bool)
                "Level" <- w255
                n200 = case shown="True" w256 {
                  tunnel: w255 -> [w276 w277]
                  frame False {
                    "Level A 2" <- w276
                  }
                  frame True {
                    "Level B 2" <- w277
                  }
                }
              }
              frame #1 {
                n201 = local write "AKNR"(FALSE ("AKNR")) -> ()
              }
            }
          }
          event "RF On": Value Change {
            # "Turn RF off and on"
            n202 = event-data() -> ()  [unwired: 1 in, 5 out]
            n203 = Boolean To (0,1)(Boolean="RF On") -> (0, 1=w323:i16)
            n204 = Number To Decimal String(number=w323) -> (decimal integer string=w321:string)  [unwired: 1 in]
            n205 = Concatenate Strings("E" ("element"), w321, "r" ("string"), w321) -> (w324:string)
            n206 = call "SerialcharWrite.vi"("VISA resource name"=w326, "write buffer"=w324) -> ("ComError"=w322:bool)  [unwired: 8 in]
            n207 = local write "COM Error"(w322) -> ()
            n208 = case shown="True" w319 {
              tunnel: "RF On" -> [w327 w328]
              frame False {
                "RFOnA2" <- w327
              }
              frame True {
                "RFOnB2" <- w328
              }
            }
          }
          event "ChLock": Value Change {
            n209 = event-data() -> ()  [unwired: 1 in, 5 out]
            n210 = local read "RF  FREQUENCY MHz  B"() -> (w334:dbl)
            n211 = local read "RF  FREQUENCY MHz A"() -> (w333:dbl)
            n212 = local read "POWER dBm A"() -> (w330:dbl)
            n213 = local read "POWER dBm B"() -> (w329:dbl)
            n214 = Subtract(x=w333, y=w334) -> (x-y=→"Freq Delta A-B":dbl)
            n215 = Subtract(x=w330, y=w329) -> (x-y=→"Amp Delta A -B":dbl)
          }
          event "Start Frequency", "Stop Frequency", "Step Time (mS)", "Step Size MHz", "Start Amplitude", "Stop Amplitude", "Leveling", "sweepdiff", "Sweep", "sweepdir", "Differential Freq", "AM Samples in Burst": Value Change {
            w335 = i16 7 ("precision (6)")
            w336 = FALSE ("use system decimal point (T)")
            # "Set up Sweep"
            n216 = event-data() -> ()  [unwired: 1 in, 5 out]
            n217 = case shown="True" "Leveling" {
              tunnel: ["Start Amplitude" w399] -> w339
              tunnel: ["Stop Amplitude" w399] -> w340
              frame False {
                w395 = T2."Enabled" ("Disabled")
                n218 = property on="Start Amplitude" class="DigNum (strict)"("DisabledEnum"=w395) -> ()  [unwired: 2 in, 2 out]
                n219 = property on="Stop Amplitude" class="DigNum (strict)"("DisabledEnum"=w395) -> ()  [unwired: 2 in, 2 out]
              }
              frame True {
                w398 = T2."Disabled and Grayed Out" ("Disabled")
                n220 = local read "POWER dBm"() -> (w399:dbl)
                n221 = local write "Start Amplitude"(w399) -> ()
                n222 = local write "Stop Amplitude"(w399) -> ()
                n223 = property on="Start Amplitude" class="DigNum (strict)"("DisabledEnum"=w398) -> ()  [unwired: 2 in, 2 out]
                n224 = property on="Stop Amplitude" class="DigNum (strict)"("DisabledEnum"=w398) -> ()  [unwired: 2 in, 2 out]
              }
            }
            n225 = Subtract(x="Stop Frequency", y="Start Frequency") -> (x-y=w375:dbl)
            n226 = Divide(x=w375, y="Step Size MHz") -> (x/y=w372:dbl)
            "Number\nof Points" <- w372
            n227 = Number To Fractional String(use system decimal point (T)=w336, number=w339, precision (6)=w335) -> (F-format string=w338:string)  [unwired: 1 in]
            n228 = Number To Fractional String(use system decimal point (T)=w336, number=w340, precision (6)=w335) -> (F-format string=w337:string)  [unwired: 1 in]
            n229 = Number To Fractional String(use system decimal point (T)=w336, number="Step Size MHz", precision (6)=w335) -> (F-format string=w378:string)  [unwired: 1 in]
            n230 = Number To Fractional String(use system decimal point (T)=w336, number="Step Time (mS)", precision (6)=w335) -> (F-format string=w376:string)  [unwired: 1 in]
            n231 = Number To Fractional String(use system decimal point (T)=w336, number="Start Frequency", precision (6)=w335) -> (F-format string=w383:string)  [unwired: 1 in]
            n232 = Number To Fractional String(use system decimal point (T)=w336, number="Stop Frequency", precision (6)=w335) -> (F-format string=w382:string)  [unwired: 1 in]
            n233 = Multiply(x="Step Time (mS)", y=w372) -> (x*y=w344:dbl)
            "Time per\nSweep (mS)" <- w344
            n234 = Not(x="sweepdir") -> (.not. x?=w354:bool)
            n235 = Boolean To (0,1)(Boolean=w354) -> (0, 1=w361:i16)
            n236 = Number To Decimal String(number=w361) -> (decimal integer string=w360:string)  [unwired: 1 in]
            n237 = Number To Decimal String(number="Sweep") -> (decimal integer string=w358:string)  [unwired: 1 in]
            n238 = Number To Decimal String(number="AM Samples in Burst") -> (decimal integer string=w348:string)  [unwired: 1 in]
            n239 = Absolute Value(x="Differential Freq") -> (abs(x)=w357:dbl)
            n240 = Number To Fractional String(use system decimal point (T)=FALSE, number=w357, precision (6)=i16 7) -> (F-format string=w351:string)  [unwired: 1 in]
            n241 = case shown="True" "sweepdiff" {
              tunnel: ["n0" ("element") w389] -> w352
              tunnel: "Differential Freq" -> [_ w391]
              frame False {
              }
              frame True {
                n242 = Greater?(x=w391, y=0.0) -> (0:w390:bool)
                n243 = case shown="False" w390 {
                  tunnel: ["n1" ("element") "n2" ("element")] -> w389
                  frame False {
                  }
                  frame True {
                  }
                }
              }
            }
            n244 = Concatenate Strings("l" ("element"), w383, "u" ("element"), w382, "s" ("element"), w378, "t" ("element"), w376, "[" ("element"), w338, "]" ("element"), w337, "^" ("element"), w360, "X" ("element"), w358, "q" ("element"), w348, "k" ("element"), w351, w352) -> (w342:string)
            n245 = Less?(x=w344, y=4.0) -> (x < y?=w341:bool)
            n246 = Greater?(x=w344, y=3600000.0) -> (0:w345:bool)
            n247 = call "SerialcharWrite.vi"("VISA resource name"=w374, "write buffer"=w342) -> ("ComError"=w384:bool)  [unwired: 8 in]
            n248 = case shown="False" w341 {
              frame False {
                n249 = property on="Sweep\nContinuously" class="Bool (strict)"("DisabledEnum"=T2."Enabled" ("Disabled")) -> ()  [unwired: 2 in, 2 out]
              }
              frame True {
                n250 = property on="Sweep\nContinuously" class="Bool (strict)"("DisabledEnum"=T2."Disabled and Grayed Out" ("Disabled")) -> ()  [unwired: 2 in, 2 out]
              }
            }
            n251 = case shown="True" w345 {
              frame False {
              }
              frame True {
                n252 = One Button Dialog(message="Sweep time is\nover 1hour.\nYou may need\n to adjust.") -> ()  [unwired: 1 in, 1 out]
              }
            }
            n253 = local write "COM Error"(w384) -> ()
          }
          event "Trigger": Value Change {
            n254 = event-data() -> ()  [unwired: 1 in, 5 out]
            n255 = case shown="2" "Trigger" {
              tunnel: [w408 "One full sweep happens after pulling down\nthe trigger signal.  It is level sensitive so\nholding down the signal repeats the sweep.\nBring high before the end of the sweep to\navoid another sweep." ("message") "Sweep Step Trigger will trigger one step in\na linear sweep or list sweep when pulled low.\nUse Step Time to debounce and make sure\nstep time is longer than your trigger pulse\nduration to avoid two steps in one pulse." ("message") "Stop All puts a \"do nothing\" hold on the\nSynthHD operating system.  It only responds\nto the Trigger and to USB.  This allows you to\ntrigger bursts of pulses or other modulations." ("message") "Quickly mutes RF power when low.  A high\nlevel restores RF power to the GUI setting." ("message") "Remove interrupts reduces jitter in modulations\nthat are timing critical.  When Trigger is pulled low\nRF is ON and Interrupts are off.  When Trigger is high\nRF is OFF and the SynthHD will respond to USB commands." ("message") "External AM Modulation is driven through the\nTrigger connector and responds to analog voltages\nbetween 0 and 1.2V.  It responds to setting stored in the\nAM look up table and cycles through each sample.  For\nbest performance set the AM frequency to 1Hz which gives\nthe maximum of 100 samples.  Set the wave shape to RAMP\nand select whether you want the response linear in dB or Volts.\n0V input will correspond with the Minimum Power setting\nand 1.2V will drive to the Peak Power setting with 100 steps\nin between.  Sample rate is roughly 22uS." ("message") "External FM Modulation is driven through the\nTrigger connector and responds to analog voltages\nbetween 0 and 1.2V.  It responds to setting stored in the\nFM control tab and cycles through each sample it creates.  For\nbest performance set the FM frequency to 1Hz which gives\nthe maximum of 100 samples.  Set the wave shape to CHIRP.\n0V input will correspond with the (neg) FM Deviation setting\nand 1.2V will drive to the (pos) Deviation setting with\n100 steps in between.  Sample rate is roughly 22uS." ("message")] -> w401
              tunnel: w400 -> [w408 _ _ _ _ _ _ _]
              frame 0, Default {
              }
              frame 1 {
              }
              frame 2 {
              }
              frame 3 {
              }
              frame 4 {
              }
              frame 5 {
                n256 = One Button Dialog(message="THIS MODE BLOCKS USB COMMUNICATIONS.\nClicking any controls while in this mode\n(with the Trigger connector pulled to ground)\nwill cause the software to lock up.  Exit this\nmode or disconnect everything from the Trigger\n connector before resuming normal operation.") -> ()  [unwired: 1 in, 1 out]
              }
              frame 8 {
              }
              frame 9 {
              }
            }
            "Specific Instructions" <- w401
            n257 = Number To Decimal String(number="Trigger") -> (decimal integer string=w405:string)  [unwired: 1 in]
            n258 = Concatenate Strings("w" ("element"), w405) -> (w407:string)
            n259 = call "SerialcharWrite.vi"("VISA resource name"=w403, "write buffer"=w407) -> ("ComError"=w404:bool)  [unwired: 8 in]
            n260 = local write "COM Error"(w404) -> ()
          }
          event "On Time (uS)", "Off Time (uS)", "# of Pulses in Burst", "Invert\nPulse": Value Change {
            # "Pulse Modulation"
            n261 = event-data() -> ()  [unwired: 1 in, 5 out]
            n262 = Add(x="On Time (uS)", y="Off Time (uS)") -> (x+y=w433:u32)
            n263 = Number To Decimal String(number="On Time (uS)") -> (decimal integer string=w428:string)  [unwired: 1 in]
            n264 = Number To Decimal String(number="Off Time (uS)") -> (decimal integer string=w429:string)  [unwired: 1 in]
            n265 = Number To Decimal String(number="# of Pulses in Burst") -> (decimal integer string=w430:string)  [unwired: 1 in]
            n266 = Multiply(x=w433, y="# of Pulses in Burst") -> (x*y=→"Duration (uS)":u32)
            n267 = Boolean To (0,1)(Boolean="Invert\nPulse") -> (0, 1=w420:i16)
            n268 = Number To Decimal String(number=w420) -> (decimal integer string=w418:string)  [unwired: 1 in]
            n269 = Concatenate Strings(":" ("string"), w418, "P" ("string"), w428, "O" ("string"), w429, "R" ("string"), w430) -> (w432:string)
            n270 = call "SerialcharWrite.vi"("VISA resource name"=w425, "write buffer"=w432) -> ("ComError"=w434:bool)  [unwired: 8 in]
            n271 = local write "COM Error"(w434) -> ()
          }
          event "Mod Tab": Value Change {
            n272 = event-data() -> ()  [unwired: 1 in, 5 out]
            n273 = local read "Modon"() -> (w436:bool)
            n274 = case shown="False" w436 {
              tunnel: w437 -> [w456 _]
              tunnel: w435 -> [w450 _]
              frame False {
                w451 = "C" ("string")
                w440 = "h1" ("write buffer")
                n275 = local read "RF  FREQUENCY MHz"() -> (w453:dbl)
                n276 = local read "POWER dBm"() -> (w445:dbl)
                n277 = Boolean To (0,1)(Boolean=w450) -> (0, 1=w452:i16)
                n278 = Not(x=w450) -> (.not. x?=w448:bool)
                n279 = Number To Decimal String(number=w452) -> (decimal integer string=w446:string)  [unwired: 1 in]
                n280 = Boolean To (0,1)(Boolean=w448) -> (0, 1=w449:i16)
                n281 = Number To Fractional String(use system decimal point (T)=FALSE, number=w445, precision (6)=i16 2) -> (F-format string=w438:string)  [unwired: 1 in]
                n282 = Number To Decimal String(number=w449) -> (decimal integer string=w447:string)  [unwired: 1 in]
                n283 = Number To Fractional String(use system decimal point (T)=FALSE, number=w453) -> (F-format string=w441:string)  [unwired: 2 in]
                n284 = Concatenate Strings("f" ("string"), w441, w440, "W" ("string"), w438, w451, w447, w440, w451, w446) -> (w455:string)
                n285 = call "SerialcharWrite.vi"("VISA resource name"=w456, "write buffer"=w455) -> ("ComError"=w457:bool)  [unwired: 8 in]
                n286 = local write "COM Error"(w457) -> ()
              }
              frame True {
              }
            }
          }
          event "Sweep\nContinuously": Value Change {
            # "Sweep Continuously"
            n287 = event-data() -> ()  [unwired: 1 in, 5 out]
            n288 = local read "Continuous AM"() -> (w459:bool)
            n289 = local read "Continuous\nPM"() -> (w461:bool)
            n290 = local read "Continuous FM"() -> (w460:bool)
            n291 = Boolean To (0,1)(Boolean="Sweep\nContinuously") -> (0, 1=w470:i16)
            n292 = case shown="True" "Sweep\nContinuously" {
              tunnel: w463 -> [_ w474]
              tunnel: ["" ("String") w473] -> w464
              frame False {
              }
              frame True {
                n293 = case shown="True" w474 {
                  tunnel: ["Sweeping Channel A" ("String") "Sweeping Channel B" ("String")] -> w473
                  frame False {
                  }
                  frame True {
                  }
                }
              }
            }
            "Swpc" <- w464
            n294 = Number To Decimal String(number=w470) -> (decimal integer string=w466:string)  [unwired: 1 in]
            n295 = Compound Arithmetic op=OR("Sweep\nContinuously", w459, w460, w461) -> (w462:bool)
            n296 = local write "Modon"(w462) -> ()
            n297 = Concatenate Strings("c" ("element"), w466, "g" ("element"), w466) -> (w467:string)
            n298 = call "SerialcharWrite.vi"("VISA resource name"=w471, "write buffer"=w467) -> ("ComError"=w465:bool)  [unwired: 8 in]
            n299 = local write "COM Error"(w465) -> ()
          }
          event "Sweep\nOnce": Value Change {
            # "Sweep Once"
            n300 = event-data() -> ()  [unwired: 1 in, 5 out]
            n301 = call "SerialcharWrite.vi"("VISA resource name"=w479, "write buffer"="g1" ("string")) -> ("ComError"=w478:bool)  [unwired: 8 in]
            n302 = local write "COM Error"(w478) -> ()
          }
          event "Continuous\nPM", "Dual Channel Mode": Value Change {
            # "Pulse Continuously"
            n303 = event-data() -> ()  [unwired: 1 in, 5 out]
            n304 = case shown="True" "Continuous\nPM" {
              tunnel: w489 -> [_ w500]
              tunnel: ["" ("String") w499] -> w490
              tunnel: "Dual Channel Mode" -> [_ w498]
              frame False {
              }
              frame True {
                n305 = case shown="True" w498 {
                  tunnel: w500 -> [w502 w505]
                  tunnel: [w501 w506] -> w499
                  frame False {
                    n306 = case shown="False" w502 {
                      tunnel: ["Modulating\nChannel A" ("String") "Modulating\nChannel B" ("String")] -> w501
                      frame False {
                      }
                      frame True {
                      }
                    }
                  }
                  frame True {
                    n307 = case shown="True" w505 {
                      tunnel: ["Modulating\nChannel A & B\n(A Controls)" ("String") "Modulating\nChannel A & B\n(B Controls)" ("String")] -> w506
                      frame False {
                      }
                      frame True {
                      }
                    }
                  }
                }
              }
            }
            "Pulsech" <- w490
            n308 = Boolean To (0,1)(Boolean="Continuous\nPM") -> (0, 1=w495:i16)
            n309 = Boolean To (0,1)(Boolean="Dual Channel Mode") -> (0, 1=w482:i16)
            n310 = local read "Sweep\nContinuously"() -> (w485:bool)
            n311 = Number To Decimal String(number=w495) -> (decimal integer string=w492:string)  [unwired: 1 in]
            n312 = local read "Continuous AM"() -> (w486:bool)
            n313 = local read "Continuous FM"() -> (w487:bool)
            n314 = Number To Decimal String(number=w482) -> (decimal integer string=w481:string)  [unwired: 1 in]
            n315 = Concatenate Strings("j" ("element"), w492, "D" ("element"), w481) -> (w493:string)
            n316 = call "SerialcharWrite.vi"("VISA resource name"=w496, "write buffer"=w493) -> ("ComError"=w491:bool)  [unwired: 8 in]
            n317 = Compound Arithmetic op=OR(w485, w486, w487, "Continuous\nPM") -> (w488:bool)
            n318 = local write "Modon"(w488) -> ()
            n319 = local write "COM Error"(w491) -> ()
          }
          event "Send Pulse\nBurst": Value Change {
            # "Send Pulse Burst"
            n320 = event-data() -> ()  [unwired: 1 in, 5 out]
            n321 = call "SerialcharWrite.vi"("VISA resource name"=w509, "write buffer"="G") -> ("ComError"=w511:bool)  [unwired: 8 in]
            n322 = local write "COM Error"(w511) -> ()
          }
          event "Continuous AM": Value Change {
            n323 = event-data() -> ()  [unwired: 1 in, 5 out]
            n324 = Boolean To (0,1)(Boolean="Continuous AM") -> (0, 1=w523:i16)
            n325 = Number To Decimal String(number=w523) -> (decimal integer string=w520:string)  [unwired: 1 in]
            n326 = case shown="True" "Continuous AM" {
              tunnel: w518 -> [_ w527]
              tunnel: ["" ("String") w526] -> w517
              frame False {
              }
              frame True {
                n327 = case shown="True" w527 {
                  tunnel: ["Modulating\nChannel A" ("String") "Modulating\nChannel B" ("String")] -> w526
                  frame False {
                  }
                  frame True {
                  }
                }
              }
            }
            "AMch" <- w517
            n328 = local read "Sweep\nContinuously"() -> (w513:bool)
            n329 = local read "Continuous\nPM"() -> (w515:bool)
            n330 = local read "Continuous FM"() -> (w514:bool)
            n331 = Concatenate Strings("A" ("element"), w520) -> (w521:string)
            n332 = call "SerialcharWrite.vi"("VISA resource name"=w524, "write buffer"=w521) -> ("ComError"=w519:bool)  [unwired: 8 in]
            n333 = local write "COM Error"(w519) -> ()
            n334 = Compound Arithmetic op=OR(w513, "Continuous AM", w514, w515) -> (w516:bool)
            n335 = local write "Modon"(w516) -> ()
          }
          event "AM Freq (Hz)", "Minimum Power (dBm)", "Peak Power(dBm)", "Wave Shape", "Linear in?": Value Change {
            # "Setup Lookup Table for AM"
            n336 = event-data() -> ()  [unwired: 1 in, 5 out]
            n337 = call "AMLUTwaveselHD2.vi"("AM Freq Hz"="AM Freq (Hz)", "Peak Power"="Peak Power(dBm)", "Min Power"="Minimum Power (dBm)", "Wave Shape"="Wave Shape", "Linear in?"="Linear in?") -> ("Waveform"=→"Waveform":dbl[], "Actual Freq"=→"Actual Freq (Hz)":dbl, "LUTsize"=→"Samples/Cycle":u8, "powerout"=w532:string)  [unwired: 7 in]
            n338 = call "SerialcharWrite.vi"("VISA resource name"=w539, "write buffer"=w532) -> ("ComError"=w540:bool)  [unwired: 8 in]
            n339 = local write "COM Error"(w540) -> ()
          }
          event "Save AM to ROM": Value Change {
            n340 = event-data() -> ()  [unwired: 1 in, 5 out]
            n341 = call "SerialcharWrite.vi"("VISA resource name"=w542, "write buffer"="@e" ("string")) -> ("ComError"=w543:bool)  [unwired: 8 in]
            n342 = local write "COM Error"(w543) -> ()
          }
          event "Read AM": Value Change {
            n343 = event-data() -> ()  [unwired: 1 in, 5 out]
            n344 = call "getAMtable2.vi"("Serial Port Select"=w544) -> ("Min dB"=w545:dbl, "Max dB"=w546:dbl, "Waveform Graph"=w547:dbl[], "AM Freq Hz"=w548:dbl)  [unwired: 5 in, 2 out]
            n345 = local write "Minimum Power (dBm)"(w545) -> ()
            n346 = local write "AM Freq (Hz)"(w548) -> ()
            n347 = local write "Waveform"(w547) -> ()
            n348 = local write "Peak Power(dBm)"(w546) -> ()
          }
          event "Save Settings\nto ROM": Value Change {
            n349 = event-data() -> ()  [unwired: 1 in, 5 out]
            n350 = call "SerialcharWrite.vi"("VISA resource name"=w549, "write buffer"="e") -> ("ComError"=w550:bool)  [unwired: 8 in]
            n351 = local write "COM Error"(w550) -> ()
          }
          event "Read\nVersion": Value Change {
            n352 = event-data() -> ()  [unwired: 1 in, 5 out]
            n353 = call "SerialCharWRtermchar.vi"("VISA resource name"=w552, "write buffer"="v0") -> ("error?"=w553:bool, "read buffer"=→"FW Version":string)  [unwired: 6 in, 1 out]
            n354 = local write "COM Error"(w553) -> ()
            n355 = case shown="False" w553 {
              tunnel: w552 -> [w556 _]
              frame False {
                n356 = call "SerialCharWRtermchar.vi"("VISA resource name"=w556, "write buffer"="v1") -> ("read buffer"=→"HW Version":string)  [unwired: 6 in, 2 out]
              }
              frame True {
              }
            }
          }
          event "Get\nTemperature": Value Change {
            n357 = event-data() -> ()  [unwired: 1 in, 5 out]
            n358 = call "SerialCharWRtermchar.vi"("VISA resource name"=w560, "write buffer"="z") -> ("read buffer"=→"Temperature":string)  [unwired: 6 in, 2 out]
          }
          event "Reference (MHz)", "Reference Select": Value Change {
            n359 = event-data() -> ()  [unwired: 1 in, 5 out]
            n360 = Number To Decimal String(number="Reference Select") -> (decimal integer string=w568:string)  [unwired: 1 in]
            n361 = case shown="0, Default" "Reference Select" {
              tunnel: [w569 "*27.0" ("write buffer") "*10.0" ("write buffer")] -> w562
              frame 0, Default {
                n362 = Number To Fractional String(use system decimal point (T)=FALSE, number="Reference (MHz)") -> (F-format string=w573:string)  [unwired: 2 in]
                n363 = Concatenate Strings("*" ("write buffer"), w573) -> (w569:string)
                n364 = property on="Reference (MHz)" class="DigNum (strict)"("DisabledEnum"=T2."Enabled" ("Disabled")) -> ()  [unwired: 2 in, 2 out]
              }
              frame 1 {
                n365 = local write "Reference (MHz)"(27.0 ("Reference (MHz)")) -> ()
                n366 = property on="Reference (MHz)" class="DigNum (strict)"("DisabledEnum"=T2."Disabled and Grayed Out" ("Disabled")) -> ()  [unwired: 2 in, 2 out]
              }
              frame 2 {
                n367 = local write "Reference (MHz)"(10.0 ("Reference (MHz)")) -> ()
                n368 = property on="Reference (MHz)" class="DigNum (strict)"("DisabledEnum"=T2."Disabled and Grayed Out" ("Disabled")) -> ()  [unwired: 2 in, 2 out]
              }
            }
            n369 = Concatenate Strings("x" ("write buffer"), w568, w562) -> (w566:string)
            n370 = call "SerialcharWrite.vi"("VISA resource name"=w564, "write buffer"=w566) -> ("ComError"=w565:bool)  [unwired: 8 in]
            n371 = local write "COM Error"(w565) -> ()
          }
          event "PLL ICP": Value Change {
            n372 = event-data() -> ()  [unwired: 1 in, 5 out]
            n373 = Number To Decimal String(number="PLL ICP") -> (decimal integer string=w582:string)  [unwired: 1 in]
            n374 = Concatenate Strings("U" ("string"), w582) -> (w584:string)
            n375 = call "SerialcharWrite.vi"("VISA resource name"=w585, "write buffer"=w584) -> ("ComError"=w586:bool)  [unwired: 8 in]
            n376 = local write "COM Error"(w586) -> ()
          }
          event "MTLD": Value Change {
            n377 = event-data() -> ()  [unwired: 1 in, 5 out]
            n378 = Boolean To (0,1)(Boolean="MTLD") -> (0, 1=w588:i16)
            n379 = Number To Decimal String(number=w588) -> (decimal integer string=w590:string)  [unwired: 1 in]
            n380 = Concatenate Strings("d" ("string"), w590) -> (w592:string)
            n381 = call "SerialcharWrite.vi"("VISA resource name"=w589, "write buffer"=w592) -> ("ComError"=w593:bool)  [unwired: 8 in]
            n382 = local write "COM Error"(w593) -> ()
          }
          event "MUX Out Select": Value Change {
            n383 = event-data() -> ()  [unwired: 1 in, 5 out]
            n384 = Number To Decimal String(number="MUX Out Select") -> (decimal integer string=w596:string)  [unwired: 1 in]
            n385 = Concatenate Strings("m" ("string"), w596) -> (w598:string)
            n386 = call "SerialcharWrite.vi"("VISA resource name"=w594, "write buffer"=w598) -> ("ComError"=w599:bool)  [unwired: 8 in]
            n387 = local write "COM Error"(w599) -> ()
          }
          event "Sync", "ChSt": Value Change {
            n388 = event-data() -> ()  [unwired: 1 in, 5 out]
            n389 = stacked-sequence {
              tunnel: w602 -> [w620 _]
              tunnel: w601 -> [w609 _]
              tunnel: w600 -> [w608 _]
              frame #0 {
                # "Load settings from SynthHD"
                # "Only send one error."
                # "Scan for Devices"
                n390 = local read "COM Error"() -> (w623:bool)
                n391 = feedback #1() -> (w625:bool)  [unwired: 1 in]
                n392 = Equal?(x=w625, y=FALSE) -> (x = y?=w628:bool)
                n393 = feedback-in #1(w623) -> ()
                n394 = Equal?(x=w623, y=TRUE) -> (x = y?=w627:bool)
                n395 = And(x=w627, y=w628) -> (x .and. y?=w629:bool)
                n396 = Or(x=w629, y="Sync") -> (x .or. y?=w622:bool)
                n397 = case shown="True" w622 {
                  tunnel: [TRUE ("Prog Chan?") FALSE ("Prog Chan?")] -> w612
                  tunnel: w608 -> [w688 _]
                  frame False {
                    n398 = case shown="False" w688 {
                      tunnel: ["B" ("Channel") "A" ("Channel")] -> w689
                      frame False {
                      }
                      frame True {
                      }
                    }
                    "Channel" <- w689
                  }
                  frame True {
                    n399 = call "getcomport.vi"() -> ("Port"=w695:string, "Device"=→"Device Under Control":string)  [unwired: 9 in, 1 out]
                    n400 = local write "Serial Port Select"(w695) -> ()
                  }
                }
                n401 = call "readparams2.vi"("Port In"=w609, "var query"=w620, "Get F&A"=TRUE, "Prog Chan?"=w612, "ChSt"=w608) -> ("RFonA"=w604:bool, "RFonB"=w603:bool, "LevA"=w605:bool, "LevB"=w606:bool, "FchA"=w619:dbl, "FchB"=w615:dbl, "ComError"=w607:bool, "AdBm"=w618:dbl, "BdBm"=w613:dbl, "NowLevel"=w617:bool, "cluster"=w611:T3, "NowFreq"=w610:dbl, "NowdBm"=w616:dbl)  [unwired: 8 in, 2 out]
                n402 = local write "Level A 2"(w605) -> ()
                n403 = local write "RFOnA2"(w604) -> ()
                n404 = local write "COM Error"(w607) -> ()
                n405 = local write "RF  FREQUENCY MHz A"(w619) -> ()
                n406 = local write "RF  FREQUENCY MHz"(w610) -> ()
                n407 = local write "POWER dBm A"(w618) -> ()
                n408 = local write "Level"(w617) -> ()
                n409 = local write "POWER dBm"(w616) -> ()
                n410 = local write "POWER dBm B"(w613) -> ()
                n411 = local write "RF  FREQUENCY MHz  B"(w615) -> ()
                n412 = local write "RFOnB2"(w603) -> ()
                n413 = local write "Level B 2"(w606) -> ()
                n414 = stacked-sequence {
                  tunnel: w611 -> [w632 w658 w682 _]
                  frame #0 {
                    n415 = Unbundle By Name(w632) -> ("[0]"=w637:dbl, "[2]"=w636:dbl, "[10]"=w631:dbl, "[30]"=w630:dbl)
                    n416 = Equal To 0?(x=w637) -> (x = 0?=w633:bool)
                    n417 = case shown="0, Default" w631 {
                      frame 0, Default {
                        n418 = property on="Reference (MHz)" class="DigNum (strict)"("DisabledEnum"=T2."Enabled" ("Disabled")) -> ()  [unwired: 2 in, 2 out]
                      }
                      frame 1 {
                        n419 = property on="Reference (MHz)" class="DigNum (strict)"("DisabledEnum"=T2."Disabled and Grayed Out" ("Disabled")) -> ()  [unwired: 2 in, 2 out]
                      }
                      frame 2 {
                        n420 = property on="Reference (MHz)" class="DigNum (strict)"("DisabledEnum"=T2."Disabled and Grayed Out" ("Disabled")) -> ()  [unwired: 2 in, 2 out]
                      }
                    }
                    n421 = local write "ChSt"(w633) -> ()
                    n422 = case shown="False" w633 {
                      tunnel: ["B" ("Channel") "A" ("Channel")] -> w634
                      frame False {
                      }
                      frame True {
                      }
                    }
                    n423 = Not Equal To 0?(x=w636) -> (x != 0?=w635:bool)
                    n424 = local write "Reference (MHz)"(w630) -> ()
                    n425 = local write "Reference Select"(w631) -> ()
                    n426 = local write "RF On"(w635) -> ()
                    n427 = local write "Channel"(w634) -> ()
                  }
                  frame #1 {
                    # "Sweep"
                    n428 = Unbundle By Name(w658) -> ("[11]"=w648:dbl, "[12]"=w647:dbl, "[13]"=w657:dbl, "[14]"=w646:dbl, "[15]"=w644:dbl, "[16]"=w643:dbl, "[17]"=w656:dbl, "[18]"=w654:dbl, "[19]"=w653:dbl, "[20]"=w649:dbl, "[21]"=w645:dbl, "[22]"=w651:dbl)
                    n429 = Equal To 0?(x=w656) -> (x = 0?=w655:bool)
                    n430 = Not Equal To 0?(x=w653) -> (x != 0?=w652:bool)
                    n431 = Not Equal To 0?(x=w645) -> (x != 0?=w650:bool)
                    n432 = local write "Differential Freq"(w654) -> ()
                    n433 = local write "Sweep\nContinuously"(w650) -> ()
                    n434 = local write "sweepdiff"(w652) -> ()
                    n435 = local write "Stop Frequency"(w647) -> ()
                    n436 = local write "Start Frequency"(w648) -> ()
                    n437 = local write "Step Size MHz"(w657) -> ()
                    n438 = local write "Step Time (mS)"(w646) -> ()
                    n439 = local write "Trigger"(w651) -> ()
                    n440 = local write "sweepdir"(w655) -> ()
                    n441 = local write "Start Amplitude"(w644) -> ()
                    n442 = local write "Stop Amplitude"(w643) -> ()
                    n443 = property on="Sweep" class="TabCtl (strict)"("Value"=w649) -> ()  [unwired: 2 in, 2 out]
                  }
                  frame #2 {
                    # "Mods"
                    n444 = Unbundle By Name(w682) -> ("[25]"=w679:dbl, "[26]"=w678:dbl, "[27]"=w677:dbl, "[28]"=w676:dbl, "[29]"=w675:dbl, "[31]"=w674:dbl, "[32]"=w673:dbl, "[33]"=w671:dbl, "[34]"=w670:dbl, "[35]"=w668:dbl, "[36]"=w667:dbl, "[37]"=w665:dbl, "[38]"=w663:dbl, "[39]"=w662:dbl, "[40]"=w661:dbl, "[41]"=w659:dbl)  [unwired: 1 out]
                    n445 = Not Equal To 0?(x=w668) -> (x != 0?=w669:bool)
                    n446 = Not Equal To 0?(x=w665) -> (x != 0?=w666:bool)
                    n447 = Not Equal To 0?(x=w662) -> (x != 0?=w664:bool)
                    n448 = Not Equal To 0?(x=w675) -> (x != 0?=w680:bool)
                    n449 = Not Equal To 0?(x=w679) -> (x != 0?=w681:bool)
                    n450 = Not Equal To 0?(x=w670) -> (x != 0?=w672:bool)
                    n451 = local write "FM Deviation (+/- Hz)"(w673) -> ()
                    n452 = local write "Fundamental\nFeedback Mode"(w669) -> ()
                    n453 = local write "FM Function"(w667) -> ()
                    n454 = local write "Invert\nPulse"(w666) -> ()
                    n455 = local write "MTLD"(w664) -> ()
                    n456 = Not Equal To 0?(x=w659) -> (x != 0?=w660:bool)
                    n457 = local write "PLL ICP"(w663) -> ()
                    n458 = local write "# of Pulses in Burst"(w676) -> ()
                    n459 = local write "Continuous\nPM"(w680) -> ()
                    n460 = local write "FM Rate (Hz)"(w674) -> ()
                    n461 = local write "MUX Out Select"(w661) -> ()
                    n462 = local write "On Time (uS)"(w678) -> ()
                    n463 = local write "Off Time (uS)"(w677) -> ()
                    n464 = local write "FM Samples in Burst"(w671) -> ()
                    n465 = local write "Continuous AM"(w681) -> ()
                    n466 = local write "Continuous FM"(w672) -> ()
                    n467 = local write "Dual Channel Mode"(w660) -> ()
                  }
                  frame #3 {
                    n468 = local read "Sweep\nContinuously"() -> (w683:bool)
                    n469 = local read "Continuous AM"() -> (w684:bool)
                    n470 = local read "Continuous\nPM"() -> (w686:bool)
                    n471 = local read "Continuous FM"() -> (w685:bool)
                    n472 = Compound Arithmetic op=OR(w683, w684, w685, w686) -> (w687:bool)
                    n473 = local write "Modon"(w687) -> ()
                  }
                }
              }
              frame #1 {
                w696 = TRUE ("Reset")
                # "reset knob memory between channels"
                # "Keep knobs working nice by\nloading with other channel value"
                n474 = flat-sequence {
                  tunnel: [w703] -> w698
                  tunnel: w698 -> [w705]
                  tunnel: [w704] -> w697
                  tunnel: w697 -> [w707]
                  frame #0 {
                    n475 = local read "Powerkn"() -> (w703:i8)
                  }
                  frame #1 {
                    n476 = feedback #2(i8 1 ("Freqkn")) -> (w704:i8)
                    n477 = feedback-in #2(w705) -> ()
                  }
                  frame #2 {
                    n478 = local write "Powerkn"(w707) -> ()
                  }
                }
                n479 = flat-sequence {
                  tunnel: [w713] -> w702
                  tunnel: w702 -> [w715]
                  tunnel: [w714] -> w701
                  tunnel: w701 -> [w717]
                  frame #0 {
                    n480 = local read "Freqkn"() -> (w713:i8)
                  }
                  frame #1 {
                    n481 = feedback #3(i8 1 ("Freqkn")) -> (w714:i8)
                    n482 = feedback-in #3(w715) -> ()
                  }
                  frame #2 {
                    n483 = local write "Freqkn"(w717) -> ()
                  }
                }
                n484 = flat-sequence {
                  tunnel: [w708] -> w700
                  tunnel: w700 -> [w710]
                  tunnel: [w709] -> w699
                  tunnel: w699 -> [w712]
                  frame #0 {
                    n485 = local read "Phasekn"() -> (w708:i8)
                  }
                  frame #1 {
                    n486 = feedback #4(i8 1 ("Freqkn")) -> (w709:i8)
                    n487 = feedback-in #4(w710) -> ()
                  }
                  frame #2 {
                    n488 = local write "Phasekn"(w712) -> ()
                  }
                }
                n489 = local write "FKNR"(w696) -> ()
                n490 = local write "PKNR"(w696) -> ()
                n491 = local write "AKNR"(w696) -> ()
              }
            }
          }
          event "Modon": Value Change {
            n492 = event-data() -> ()  [unwired: 1 in, 5 out]
            n493 = case shown="False" "Modon" {
              tunnel: w718 -> [w721 _]
              frame False {
                w723 = FALSE ("Sweep\nContinuously")
                # "Turn off all mods"
                n494 = call "SerialcharWrite.vi"("VISA resource name"=w721, "write buffer"="g0c0/0j0A0" ("string")) -> ("ComError"=w722:bool)  [unwired: 8 in]
                n495 = local write "Sweep\nContinuously"(w723) -> ()
                n496 = local write "Continuous AM"(w723) -> ()
                n497 = local write "Continuous\nPM"(w723) -> ()
                n498 = local write "Continuous FM"(w723) -> ()
                n499 = local write "COM Error"(w722) -> ()
              }
              frame True {
                n500 = local write "Modon"(FALSE ("Modon")) -> ()
              }
            }
          }
          event "FM Rate (Hz)", "FM Deviation (+/- Hz)", "FM Samples in Burst", "FM Function": Value Change {
            w734 = 16.0 ("y")
            n501 = event-data() -> ()  [unwired: 1 in, 5 out]
            n502 = Divide(x=u16 464 ("y"), y="FM Rate (Hz)") -> (x/y=w737:dbl)
            n503 = Number To Decimal String(number="FM Function") -> (decimal integer string=w740:string)  [unwired: 1 in]
            n504 = Number To Decimal String(number="FM Deviation (+/- Hz)") -> (decimal integer string=w745:string)  [unwired: 1 in]
            n505 = Number To Decimal String(number="FM Samples in Burst") -> (decimal integer string=w742:string)  [unwired: 1 in]
            n506 = Number To Decimal String(number="FM Rate (Hz)") -> (decimal integer string=w748:string)  [unwired: 1 in]
            n507 = Round Toward -Infinity(1:w737) -> (0:w736:dbl)
            n508 = Multiply(x=w736, y=w734) -> (x*y=w735:dbl)
            n509 = Add(x=w735, y=w734) -> (x+y=w733:dbl)
            n510 = Multiply(x="FM Rate (Hz)", y=w733) -> (x*y=w731:dbl)
            n511 = Concatenate Strings("<" ("string"), w748, ">" ("string"), w745, "," ("string"), w742, ";" ("string"), w740) -> (w750:string)
            n512 = call "SerialcharWrite.vi"("VISA resource name"=w751, "write buffer"=w750) -> ("ComError"=w752:bool)  [unwired: 8 in]
            n513 = Divide(x=1000000.0, y=w731) -> (x/y=w729:dbl)
            n514 = Round Toward -Infinity(1:w729) -> (0:w728:dbl)
            n515 = local write "COM Error"(w752) -> ()
            n516 = In Range and Coerce(upper limit=100.0, x=w728, lower limit=0.0) -> (coerced(x)=→"FM Samples / Cycle":dbl)  [unwired: 1 out]
          }
          event "Continuous FM": Value Change {
            n517 = event-data() -> ()  [unwired: 1 in, 5 out]
            n518 = Boolean To (0,1)(Boolean="Continuous FM") -> (0, 1=w761:i16)
            n519 = Number To Decimal String(number=w761) -> (decimal integer string=w760:string)  [unwired: 1 in]
            n520 = case shown="True" "Continuous FM" {
              tunnel: w755 -> [_ w768]
              tunnel: ["" ("String") w767] -> w753
              frame False {
              }
              frame True {
                n521 = case shown="True" w768 {
                  tunnel: ["Modulating\nChannel A" ("String") "Modulating\nChannel B" ("String")] -> w767
                  frame False {
                  }
                  frame True {
                  }
                }
              }
            }
            "FMch" <- w753
            n522 = local read "Sweep\nContinuously"() -> (w756:bool)
            n523 = local read "Continuous AM"() -> (w757:bool)
            n524 = local read "Continuous\nPM"() -> (w758:bool)
            n525 = Concatenate Strings("/" ("string"), w760) -> (w763:string)
            n526 = call "SerialcharWrite.vi"("VISA resource name"=w764, "write buffer"=w763) -> ("ComError"=w765:bool)  [unwired: 8 in]
            n527 = local write "COM Error"(w765) -> ()
            n528 = Compound Arithmetic op=OR(w756, w757, "Continuous FM", w758) -> (w759:bool)
            n529 = local write "Modon"(w759) -> ()
          }
          event "Read Settings\nFrom SynthHD": Value Change {
            n530 = event-data() -> ()  [unwired: 1 in, 5 out]
            n531 = call "SerialCharWriteandRead.vi"("VISA resource name"=w771, "write buffer"="?") -> ("error?"=w772:bool, "read buffer"=→"read buffer":string)  [unwired: 5 in, 2 out]
            n532 = local write "COM Error"(w772) -> ()
          }
          event "Read Registers": Value Change {
            n533 = event-data() -> ()  [unwired: 1 in, 5 out]
            n534 = call "SerialCharWriteandRead.vi"("VISA resource name"=w775, "write buffer"="H?") -> ("error?"=w777:bool, "read buffer"=→"Hex buf":string)  [unwired: 5 in, 2 out]
            n535 = local write "COM Error"(w777) -> ()
          }
          event "stop": Value Change {
            n536 = event-data() -> ()  [unwired: 1 in, 5 out]
          }
          event Panel Close? {
            w781 = TRUE ("Discard?")
            n537 = event-data() -> ("VIRef"=w782:refnum<vi>)  [unwired: 1 in]
            n538 = Close Reference(reference=w782) -> ()  [unwired: 1 in, 1 out]
            n539 = event-data("Discard?"=w781) -> ()  [unwired: 1 in, 1 out]
          }
          event Timeout {
            n540 = event-data() -> ()  [unwired: 1 in, 2 out]
            n541 = case shown="True" w783 {
              tunnel: w784 -> [_ w786]
              frame False {
              }
              frame True {
                w785 = T4 128 items=["Flush Receive Buffer"=16, "Write Transmit Buffer to Device"=32, "Flush Receive Buffer (No I/O)"=64, "Flush Transmit Buffer"=128] ("Mask")
                w788 = T4 64 items=["Flush Receive Buffer"=16, "Write Transmit Buffer to Device"=32, "Flush Receive Buffer (No I/O)"=64, "Flush Transmit Buffer"=128] ("Mask")
                n542 = VISA Flush I/O Buffer(VISA resource name=w786, mask (16)=w788) -> (error out=w787:errorcluster)  [unwired: 1 in, 1 out]
                n543 = VISA Flush I/O Buffer(VISA resource name=w786, mask (16)=w785, error in (no error)=w787) -> ()  [unwired: 2 out]
              }
            }
          }
          event "Get Phase\nLock Status": Value Change {
            n544 = event-data() -> ()  [unwired: 1 in, 5 out]
            n545 = case shown="False" "Get Phase\nLock Status" {
              tunnel: [FALSE w797] -> w791
              tunnel: w790 -> [_ w793]
              frame False {
              }
              frame True {
                n546 = call "SerialCharWRtermchar.vi"("VISA resource name"=w793, "write buffer"="p") -> ("error?"=w794:bool, "read buffer"=w795:string)  [unwired: 6 in, 1 out]
                n547 = Fract/Exp String To Number(string=w795) -> (number=w799:dbl)  [unwired: 3 in, 1 out]
                n548 = local write "COM Error"(w794) -> ()
                n549 = Not Equal?(x=0.0, y=w799) -> (x != y?=w797:bool)
              }
            }
            "Lock" <- w791
          }
          event "Re-Init Settings\nto Default": Value Change {
            n550 = event-data() -> ()  [unwired: 1 in, 5 out]
            n551 = stacked-sequence {
              tunnel: w800 -> [w802 _ _ w807]
              frame #0 {
                # "Re-init firmware"
                n552 = call "SerialcharWrite.vi"("VISA resource name"=w802, "write buffer"="|w") -> ()  [unwired: 8 in, 1 out]
              }
              frame #1 {
                # "wait for firmware reboot"
                n553 = Wait (ms)(milliseconds to wait=u32 2000) -> ()  [unwired: 1 out]
              }
              frame #2 {
                n554 = One Button Dialog(message="Re-init complete.  Please\nclick Scan Devices.") -> ()  [unwired: 1 in, 1 out]
              }
              frame #3 {
                # "Program factory\ndefaults"
                n555 = call "createtable.vi"() -> ("tab output"=w805:string)  [unwired: 11 in]
                n556 = call "AMLUTwaveselHD2.vi"() -> ("powerout"=w806:string)  [unwired: 12 in, 3 out]
                n557 = Concatenate Strings(w806, "@e" ("string"), w805, "C1E0r0f1000.0a18612C0E1r1f1000.0a18612e" ("write buffer")) -> (w808:string)
                n558 = call "SerialcharWrite.vi"("VISA resource name"=w807, "write buffer"=w808) -> ()  [unwired: 8 in, 1 out]
              }
            }
          }
        }
      }
    }
    frame #3 {
      n559 = case shown="False" w811 {
        frame False {
          n560 = Open VI Reference(vi path=path "SynthHD_2_0a.vi") -> (vi reference=w813:refnum<vi>)  [unwired: 5 in, 1 out]
          n561 = invoke class="VI" method="FP.Close"(reference=w813) -> ()  [unwired: 2 in, 3 out]
        }
        frame True {
        }
      }
    }
  }
  n562 = control-ref of="This VI"() -> (w2:refnum<vi>)
  n563 = register-events "Register For Events"(w2) -> (reference out=w3:refnum<event-registration>)  [unwired: 2 in, 1 out]
  n564 = local write "Specific Instructions"(w1) -> ()
